vi "RestDataList.vi"(8 "error in (no error)":errorcluster caption="错误输入（无错误）", 11 "real report 3":refnum<vi>) -> (0 "error out":errorcluster caption="错误输出", 3 "引用输出":refnum<vi>)   [LabVIEW 2018]
uses:
  <vilib>/Utility/miscctls.llb/LVRowAndColumnTypeDef.ctl
panel:
  in  "real report 2":i32(listbox) caption="real report"
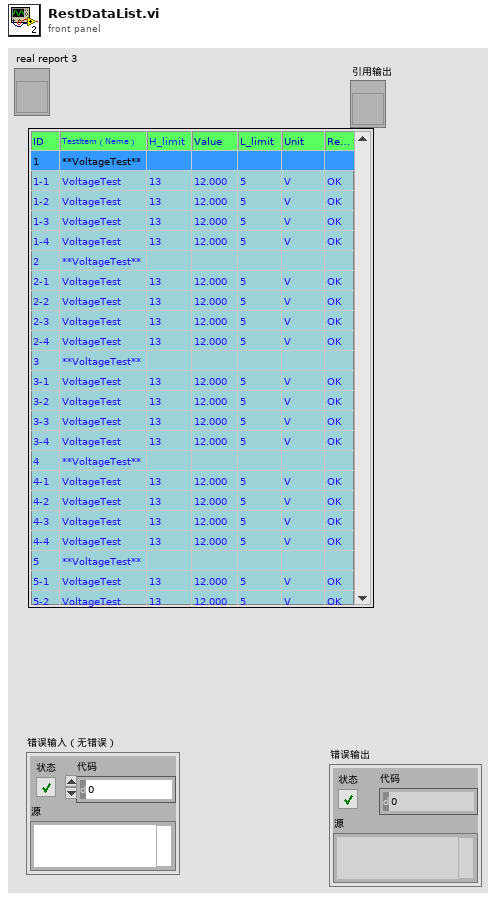
[diagram p1: front panel]
types:
  T1 = typedef "LVRowAndColumnTypeDef.ctl" = cluster{"Row":i32, "Column":i32}
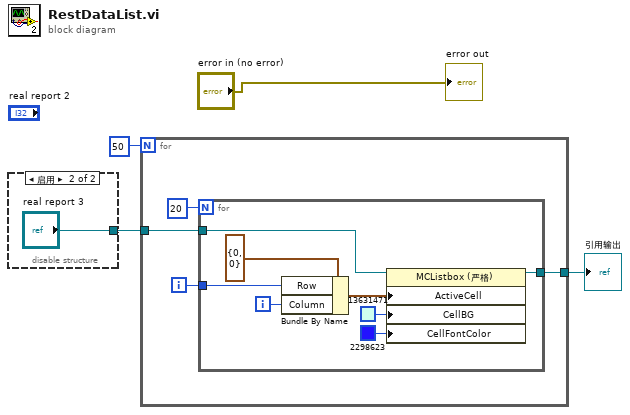
[diagram p0: block diagram]
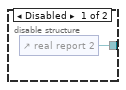
[diagram p2: hidden frame]
diagram:
  n1 = disable-structure shown="启用" {
    disable-tunnel: [w5 "real report 3"] -> w4
    frame Disabled {
      n2 = control-ref of="real report 2"() -> (w5:refnum<vi>)
    }
    frame Enabled {
    }
  }
  n3 = for {
    N: 50 -> [_]
    tunnel: w4 -> [w10]
    tunnel: [w7] -> w2
    i -> [w9]
    n4 = for {
      N: 20 -> [_]
      tunnel: w10 -> [w18]
      tunnel: w9 -> [w15]
      tunnel: [w11] -> w7
      i -> [w14]
      n5 = Bundle By Name(cluster=T1 {"Row"=0, "Column"=0} ("活动单元格:活动单元格"), "Row"=w15, "Column"=w14) -> (w16:T1)
      n6 = property class="MCListbox (严格)"(reference=w18, "ActiveCell"=w16, "CellBG"=u32 13631471, "CellFontColor"=u32 2298623) -> (reference out=w11:refnum<vi>)  [unwired: 1 in, 1 out]
    }
  }
  "引用输出" <- w2
  "error out" <- "error in (no error)"
